vi "UI(Launcher).vi"(8 "error in":errorcluster) -> (0 "error out":errorcluster)   [LabVIEW 2017, in "UI.lvlib"]
doc: "The Queued Message Handler of a Worker."
uses:
  UI.lvlib
  <userlib>/_NEVSTOP/Communicable State Machine(CSM)/_Support/Priority Queue/Priority Queue.lvclass/Priority Queue.ctl
  _support/Settings.ctl
  Acquisition/_support/Hardware Configuration.ctl
  Acquisition/_support/Signal Type.ctl
  Logging/_support/Logging Configuration.ctl
  _support/Control Refs.ctl
  _support/UI State.ctl
  a36ec0c4-7f1b-4461-99c1-16b6f02c0371.vi
  1af51285-6659-428e-9c15-de70f1a207c9.vi
  1756710f-d813-4077-a3f9-6f06171a4225.vi
  242d01f8-d211-4c25-bb6c-8191a2acbe42.vi
  <userlib>/_NEVSTOP/Communicable State Machine(CSM)/_Polymophic/Add State(s) to Queue By BOOL(Element).vi
  <userlib>/_NEVSTOP/Communicable State Machine(CSM)/_Polymophic/Build No-Reply Asynchronous Message with Arguments.vi
  <userlib>/_NEVSTOP/Communicable State Machine(CSM)/_Support/CSMQ/_Obtain CSMQ.vi
  <userlib>/_NEVSTOP/Communicable State Machine(CSM)/_Support/FGV-BroadcastRegistry/Cache-Broadcast Registry Search Result.vi
  <userlib>/_NEVSTOP/Communicable State Machine(CSM)/_Support/CSMQ/_Create Resp Queue.vi
  <userlib>/_NEVSTOP/Communicable State Machine(CSM)/_Support/CSMQ/_Unlock CSMQ.vi
  <userlib>/_NEVSTOP/Communicable State Machine(CSM)/_Support/CSMQ/_Lock State CSMQ.vi
  <userlib>/_NEVSTOP/Communicable State Machine(CSM)/_Support/CSMQ/_Release CSMQ.vi
  <userlib>/_NEVSTOP/Communicable State Machine(CSM)/AdvanceAPI/CSM - Make String Arguments Safe.vi
  <userlib>/_NEVSTOP/Communicable State Machine(CSM)/addons/API-String-Arugments-Support/_Support/Query Data as API String Arguments(variant).vi
  <userlib>/_NEVSTOP/Communicable State Machine(CSM)/_Support/Message/Parse State with Arguments String.vi
  <userlib>/_NEVSTOP/Communicable State Machine(CSM)/_Support/CSMQ/_Input Name to CSM Mode.vi
  <userlib>/_NEVSTOP/Communicable State Machine(CSM)/_Support/Priority Queue/Not a Refnum.vi
  <userlib>/_NEVSTOP/Communicable State Machine(CSM)/Utility/uuid.vi
  <userlib>/_NEVSTOP/Communicable State Machine(CSM)/AdvanceAPI/CSM - Keywords.vi
  <userlib>/_NEVSTOP/Communicable State Machine(CSM)/_Support/GlobalEvent/FGV-GlobalEventRef.vi
  <userlib>/_NEVSTOP/Communicable State Machine(CSM)/_Support/CSMQ/_CSMQFGV.vi
  <userlib>/_NEVSTOP/Communicable State Machine(CSM)/_Support/CSMQ/_Dequeue CSMQ.vi
  <userlib>/_NEVSTOP/Communicable State Machine(CSM)/_Support/CSMQ/_Enqueue CSMQ.vi
  <userlib>/_NEVSTOP/Communicable State Machine(CSM)/_Support/GlobalEvent/FGV-StatusChangeEventRef.vi
  <userlib>/_NEVSTOP/Communicable State Machine(CSM)/_Support/FGV-BroadcastRegistry/global-Broadcast Cache Change Flag.vi
  <userlib>/_NEVSTOP/Communicable State Machine(CSM)/_Support/FGV-BroadcastRegistry/FGV-BroadcastRegistry.vi
  <userlib>/_NEVSTOP/Communicable State Machine(CSM)/addons/API-String-Arugments-Support/_Support/Data To API String Arguments.vi
  <userlib>/_NEVSTOP/Communicable State Machine(CSM)/addons/INI-Static-Variable-Support/LabVIEW-Config/Write Key (String).vi
  <userlib>/_NEVSTOP/Communicable State Machine(CSM)/addons/API-String-Arugments-Support/_Support/Convert API String Arguments to Data(variant).vi
  <userlib>/_NEVSTOP/Communicable State Machine(CSM)/addons/API-String-Arugments-Support/_Support/Data To SingleElementsArray_with_itself_csm.vi
  <userlib>/_NEVSTOP/Communicable State Machine(CSM)/addons/MassData-Parameter/_support/FGV-MassData.vi
  _support/Settings Dialog.vi
  Acquisition/Acquisition.lvlib
  Logging/Logging.lvlib
  <userlib>/_NEVSTOP/Communicable State Machine(CSM)/Communicable State Machine.lvlib
  <userlib>/_NEVSTOP/Communicable State Machine(CSM)/addons/MassData-Parameter/CSM MassData Parameter Support.lvlib
  <userlib>/_NEVSTOP/Communicable State Machine(CSM)/addons/INI-Static-Variable-Support/INI-Static-Variable-Support.lvlib
  <userlib>/_NEVSTOP/Communicable State Machine(CSM)/addons/INI-Static-Variable-Support/LabVIEW-Config/LabVIEW-Config.lvlib
  Algorithm/Algorithm.lvlib
panel:
  out "State History":string
  out "Data":waveform(dbl)[](graph)
  in  "Settings":bool
  in  "Start":bool
  in  "Stop":bool
  out "Status":string
  in  "Exit":bool
  # "Continuous Measurement and Data Logger - CSM Version"
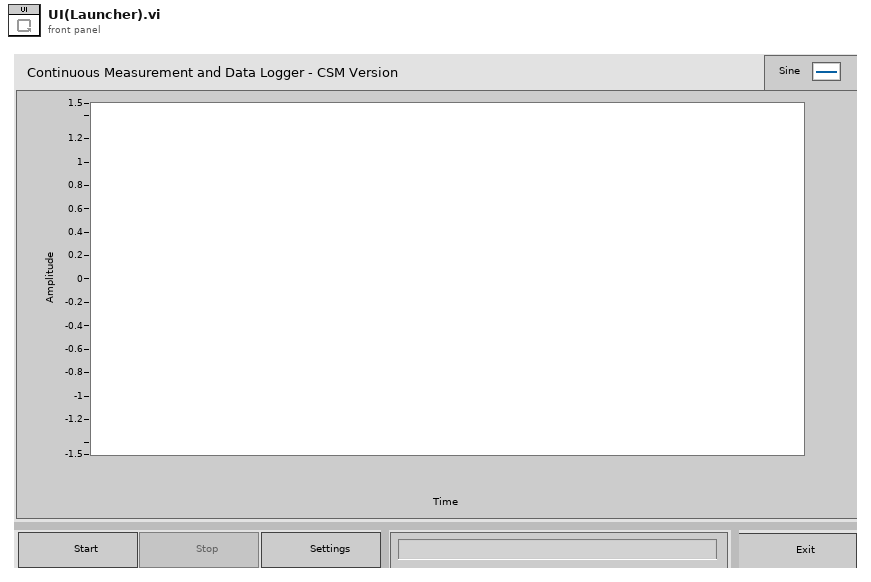
[diagram p1: front panel]
types:
  T1 = enum32{"Invalid", "Standard", "Closed", "Hidden", "Minimized", "Maximized"}
  T2 = enum32{"invalid app kind", "Development System", "Run Time System", "Student Edition", "Embedded LabVIEW", "Evaluation", "Custom"}
  T3 = typedef "UI.lvlib/UI State.ctl" = enum16{"Idle", "Acquiring and Logging", "Waiting for Exit", "Waiting for Exit (Acq Stopped)", "Waiting for Exit (Log Stopped)", "Waiting for Stop", "Waiting for Stop (Acq Stopped)", "Waiting for Stop (Log Stopped)"}
  T4 = typedef "UI.lvlib/Settings.ctl" = cluster{"Hardware":T5, "Logging":T7}
  T5 = typedef "Acquisition.lvlib/Hardware Configuration.ctl" = cluster{"Resource":string, "SignalType":T6}
  T6 = typedef "Acquisition.lvlib/Signal Type.ctl" = enum16{"Sine Wave", "Square with Noise"}
  T7 = typedef "Logging.lvlib/Logging Configuration.ctl" = cluster{"BasePath":path}
  T8 = typedef "UI.lvlib/Control Refs.ctl" = cluster{"Start Ref":refnum<vi>, "Stop Ref":refnum<vi>, "Settings Ref":refnum<vi>, "Exit Ref":refnum<vi>, "Status Ref":refnum<vi>, "Data Ref":refnum<vi>}
  T9 = cluster{"Core":cluster{"Current VI Reference":refnum<vi>, "Close Panel on Exit?":bool}, "Config":T4, "UI Refs":T8, "State":T3}
  T10 = cluster{"Current VI Reference":refnum<vi>, "Close Panel on Exit?":bool}
  T11 = typedef "LabVIEW-Config.lvlib/Config.ctl" = cluster{"Path":path, "Lines":string[], "Tokens":enum8{"comment", "section", "key"}[], "Modified?":bool}
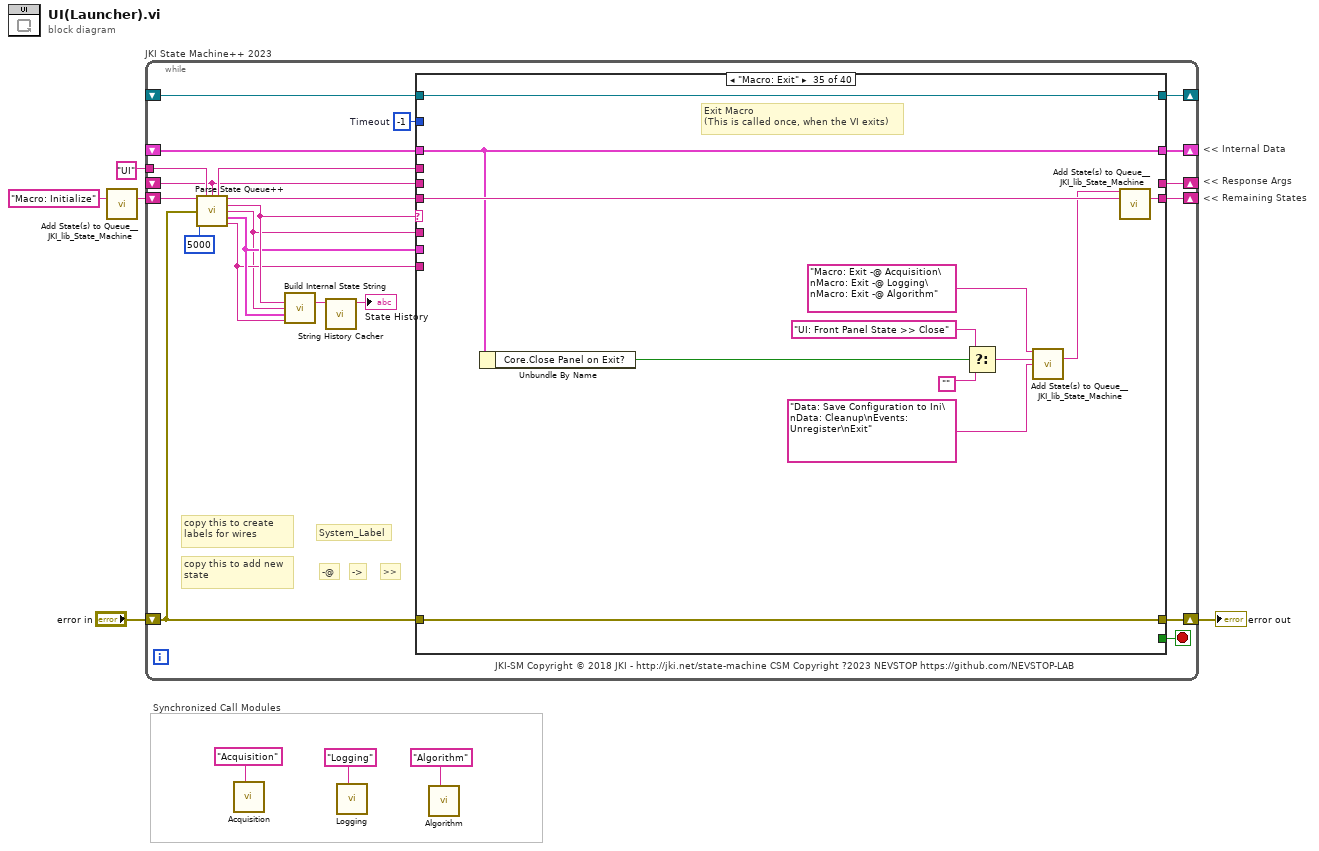
[diagram p0: block diagram]
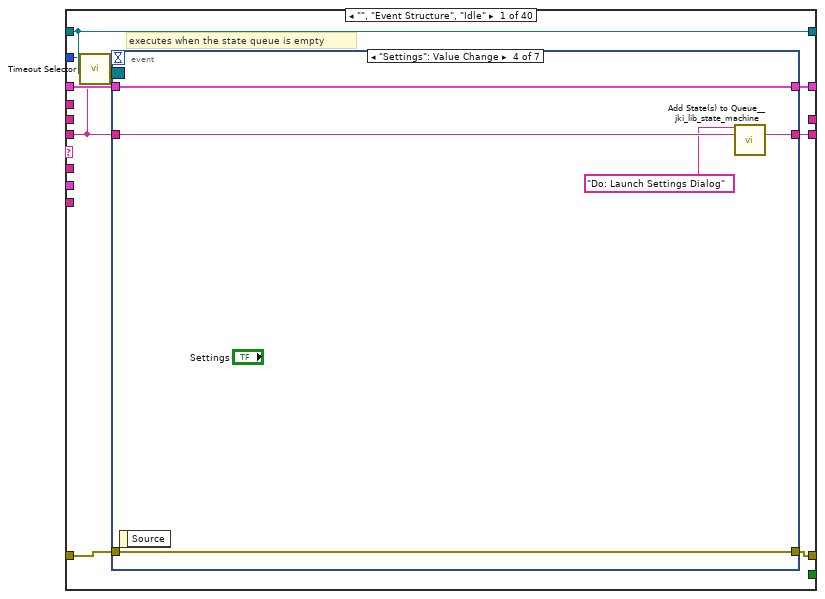
[diagram p2: hidden frame]
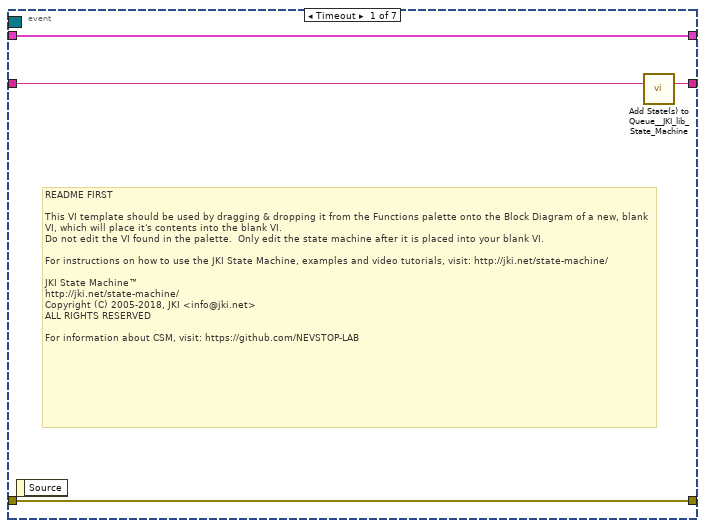
[diagram p3: hidden frame]
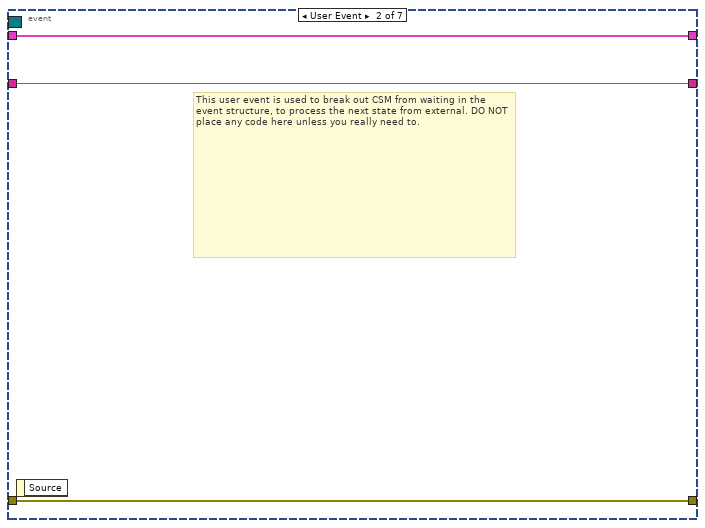
[diagram p4: hidden frame]
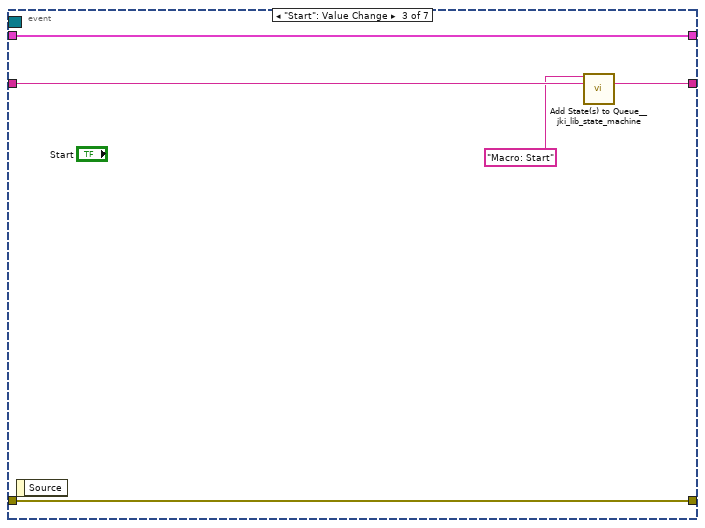
[diagram p5: hidden frame]
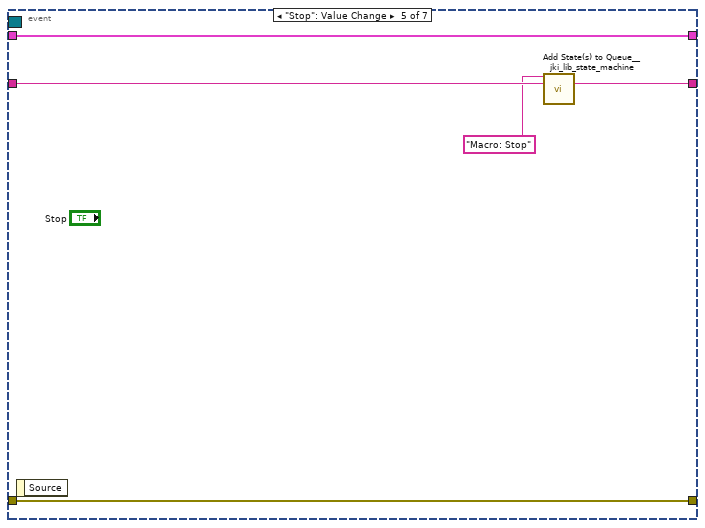
[diagram p6: hidden frame]
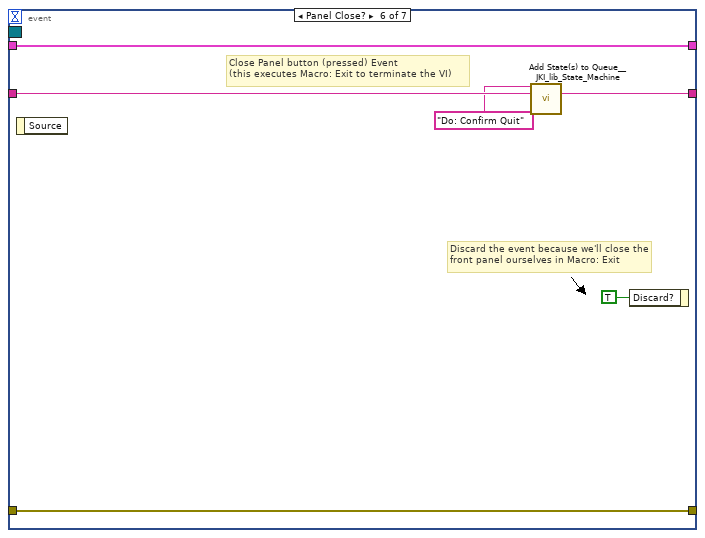
[diagram p7: hidden frame]
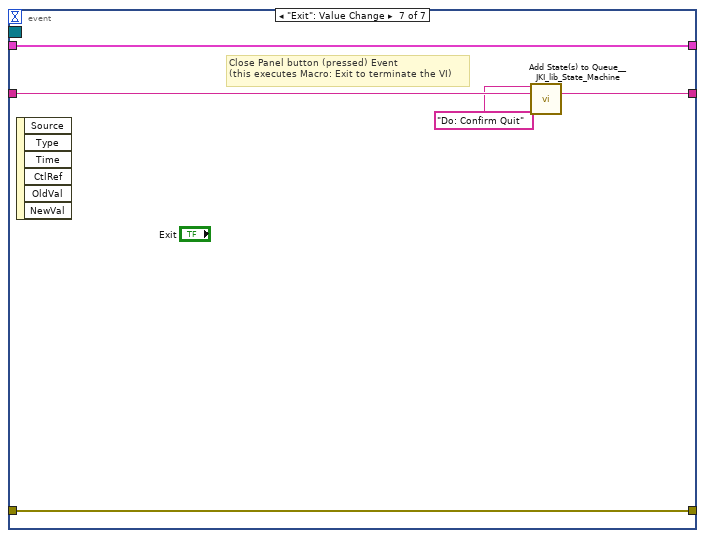
[diagram p8: hidden frame]
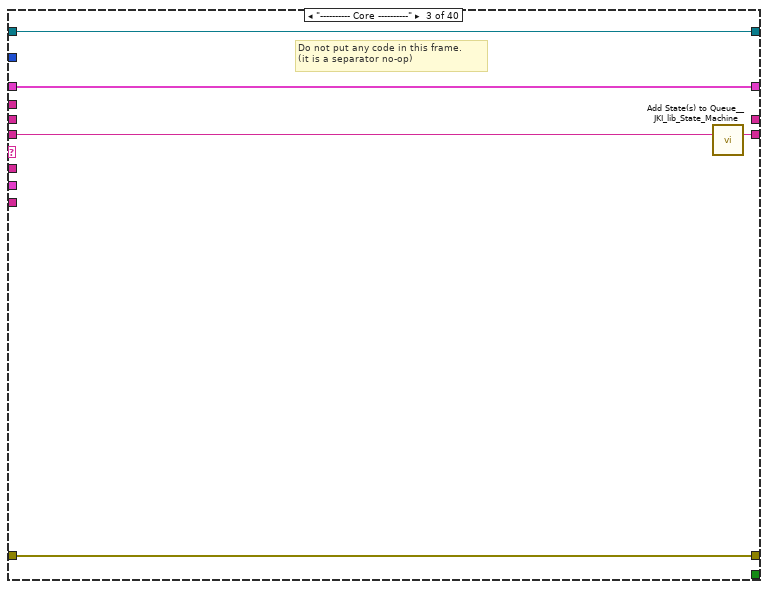
[diagram p10: hidden frame]
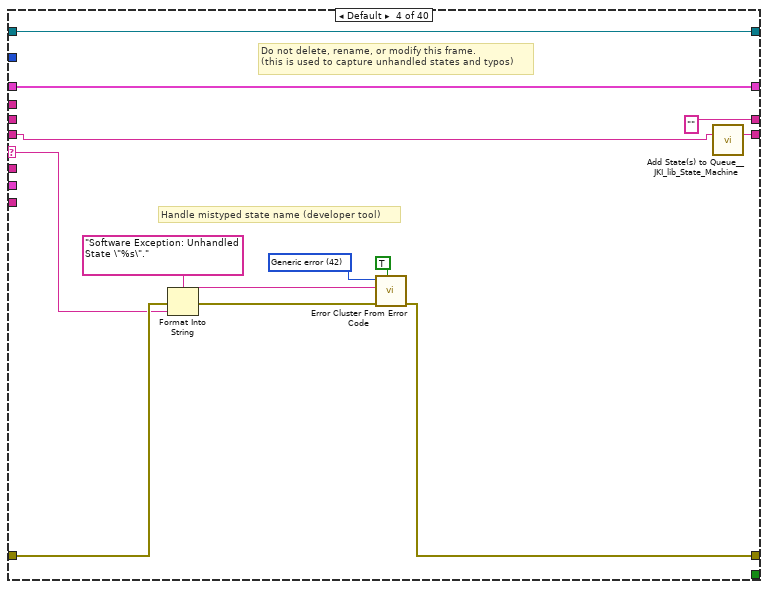
[diagram p11: hidden frame]
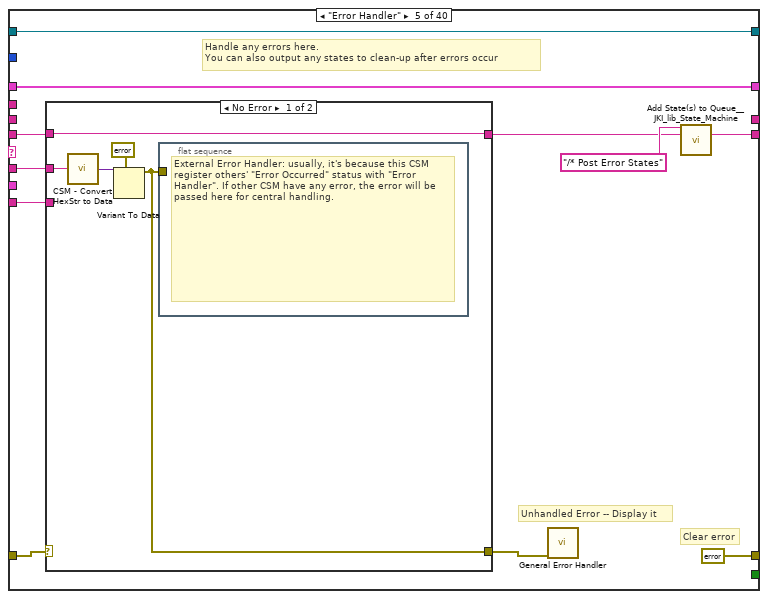
[diagram p12: hidden frame]
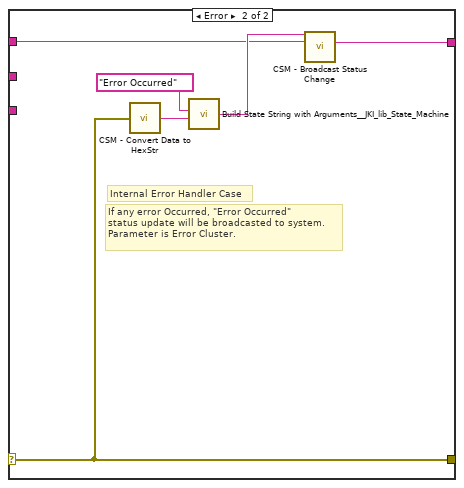
[diagram p13: hidden frame]
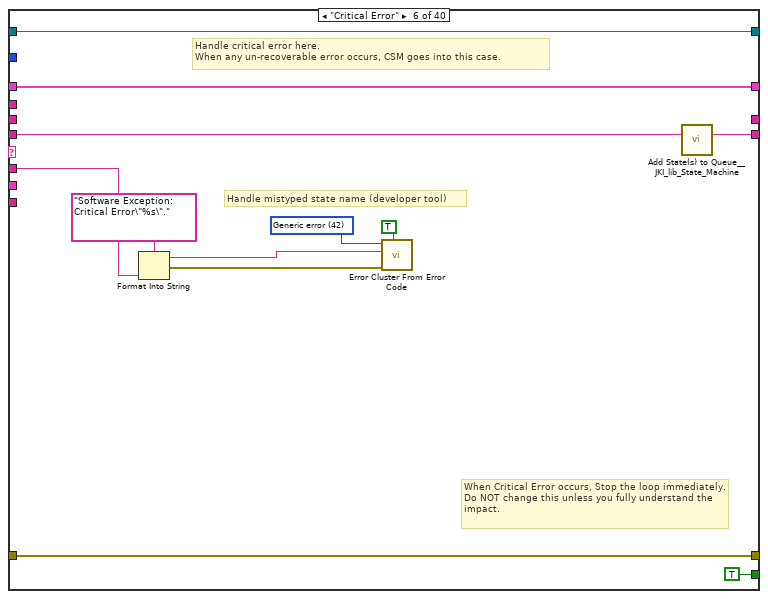
[diagram p14: hidden frame]
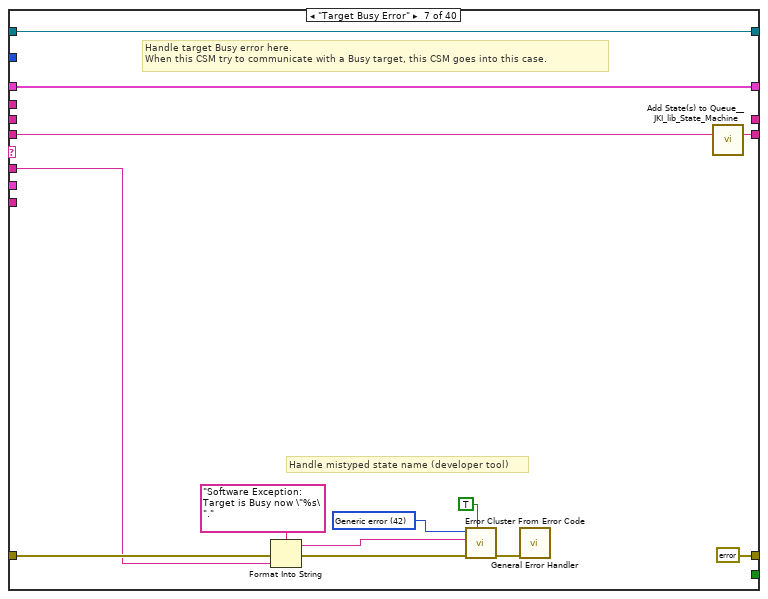
[diagram p15: hidden frame]
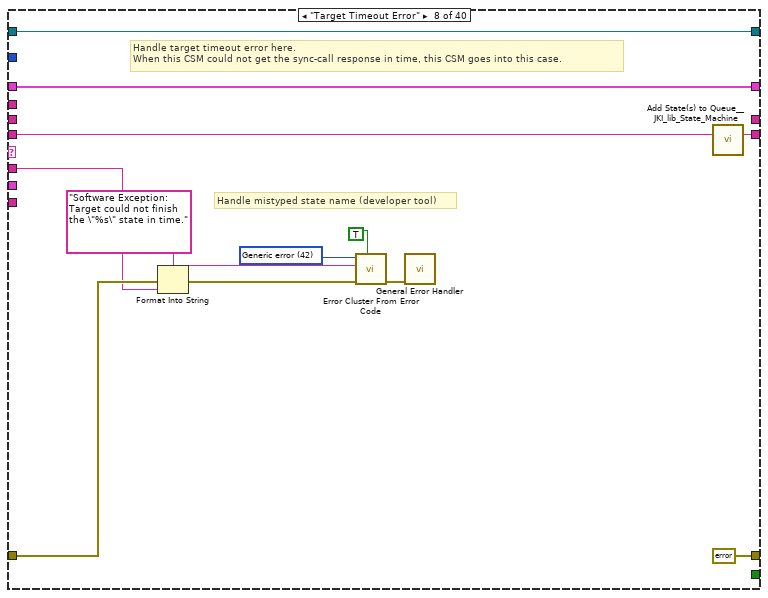
[diagram p16: hidden frame]
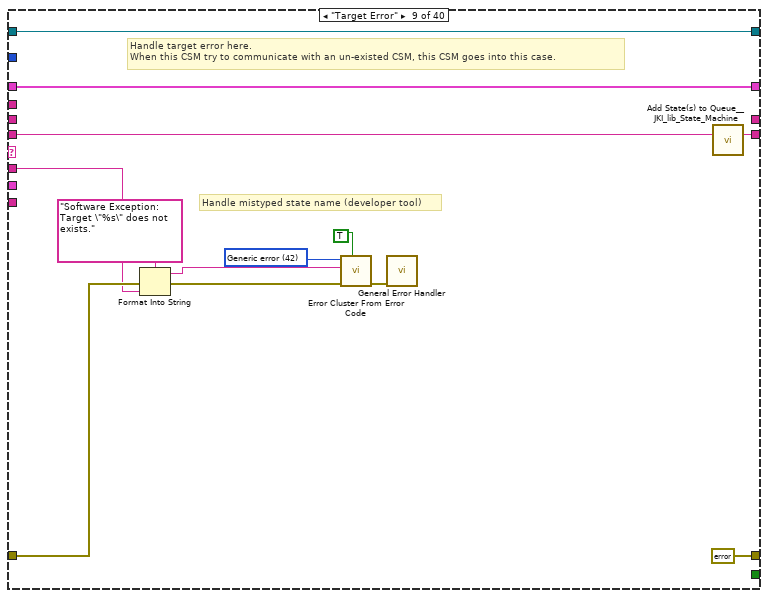
[diagram p17: hidden frame]
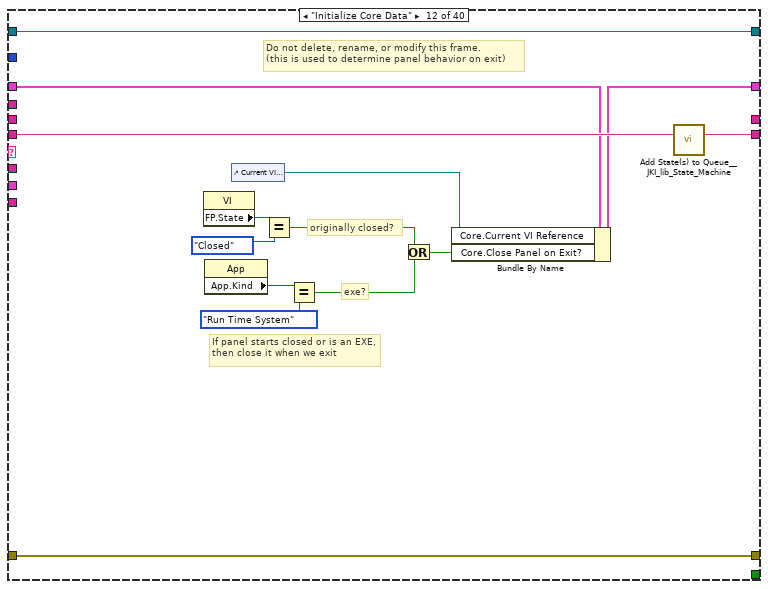
[diagram p20: hidden frame]
diagram:
  # "Synchronized Call Modules"
  # "<< Internal Data"
  # "<< Response Args"
  # "<< Remaining States"
  n1 = call <vilib>:"Add State(s) to Queue__JKI_lib_State_Machine.vi"("State(s) in (\"\")"="Macro: Initialize") -> ("States Out"=w6:string)  [unwired: 14 in]
  n2 = while "JKI State Machine++ 2023" {
    shift-right: [w25] -> _
    shift-left: _ -> [w24]
    shift-right: [w28] -> w4
    shift-left: "error in" -> [w22]
    shift-right: [w27] -> _
    shift-left: w6 -> [w29]
    tunnel: "UI" ("Name(\"\" to use uuid)") -> [w17]
    shift-right: [w20] -> _
    shift-left: _ -> [w10]
    shift-right: [w19] -> _
    shift-left: _ -> [w18]
    stop <- w26 stop-if-true
    w23 = -1  # Timeout
    # "JKI-SM Copyright © 2018 JKI - http://jki.net/state-machine CSM Copyright ?2023 NEVSTOP https://github.com/NEVSTOP-LAB"
    # "copy this to add new state"
    # ">>"
    # "->"
    # "-@"
    # "copy this to create labels for wires"
    # "System_Label"
    n3 = call <userlib>:"Parse State Queue++.vi"("State Queue"=w29, "Name(\"\" to use uuid)"=w17, "Response Arguments"=w10, "Error In (no error)"=w22, "Response Timeout(5000ms)"=5000 ("Response Timeout(1000ms)")) -> ("Name Used"=w11:string, "Remaining States"=w30:string, "Current State"=w14:string, "Arguments"=w9:string, ">> Response Source Message >>"=w13:cluster{"State":string, "Arguments":string}, ">> Source CSM >>"=w12:string)  [unwired: 5 in]
    n4 = call <userlib>:"Build Internal State String.vi"("State"=w14, "Arguments (\"\")"=w9, ">> Response Source Message >>"=w13, "Source (\"\")"=w12) -> ("State with Arguments"=w15:string)  [unwired: 11 in]
    n5 = call <userlib>:"String History Cacher.vi"("String"=w15) -> ("String Cache"=→"State History":string)  [unwired: 10 in]
    n6 = case shown="\"Macro: Exit\"" w14 {
      selector: w14 -> [_ _ _ w84 _ _ _ _ _ _ _ _ _ _ _ _ _ _ _ _ _ _ _ _ _ _ _ _ _ _ _ _ _ _ _ _ _ _ _ _]
      tunnel: w30 -> [w31 w75 w81 w88 w98 w126 w131 w149 w162 w170 w174 w189 w196 w201 w216 w220 w240 w258 w265 w272 w277 w283 w287 w293 w310 w321 w333 w341 w357 w429 w434 w441 w447 w462 w483 w488 w494 w505 w517 w532]
      tunnel: w9 -> [_ _ _ _ w96 w119 w133 w145 w158 _ _ _ _ _ _ _ _ w256 w262 _ _ _ _ _ _ _ _ w336 w351 w426 _ _ _ _ _ _ w489 _ _ _]
      tunnel: w24 -> [w38 w74 w78 w86 w104 w127 w135 w147 w160 w169 w173 w182 w194 w198 _ w222 w232 w255 w263 w267 w274 w282 w286 w290 w296 w311 w323 w339 w353 w428 w431 w438 w450 w458 w480 w485 w491 w500 w516 w527]
      tunnel: [w37 w76 w79 w90 errorcluster {"status"=FALSE, "code"=0, "source"=""} ("error out") w128 errorcluster {"status"=FALSE, "code"=0, "source"=""} ("error out") errorcluster {"status"=FALSE, "code"=0, "source"=""} ("error out") errorcluster {"status"=FALSE, "code"=0, "source"=""} ("error out") w171 w175 w186 w193 w199 w202 w223 w241 w253 w261 w268 w275 w278 w285 w291 w308 w322 w334 w337 w354 w423 w432 w439 w453 w466 w481 w486 w492 w497 w520 w525] -> w28
      tunnel: w22 -> [w36 w76 w79 w89 w102 w128 w137 w150 w163 w171 w175 w186 w193 w199 w203 w223 w241 _ _ w269 w275 _ w288 w291 w308 w322 w334 w338 w355 _ w432 w439 w453 w466 w481 w486 w492 w498 w520 w526]
      tunnel: [w39 w75 w80 w87 w100 w125 w136 w148 w161 w170 w174 w188 w195 w200 w215 w219 w240 w258 w265 w271 w276 w283 w287 w292 w309 w321 w333 w340 w356 w429 w433 w440 w448 w463 w482 w487 w493 w504 w518 w523] -> w27
      tunnel: [_ _ _ _ _ TRUE _ _ _ _ _ _ TRUE _ _ _ _ _ _ _ _ _ _ _ _ _ _ _ _ _ _ _ _ _ _ _ _ _ _ _] -> w26
      tunnel: [w35 w74 w78 w86 w104 w127 w135 w147 w160 w169 w173 w187 w194 w198 w214 w222 w232 w254 w259 w267 w274 w282 w286 w290 w295 w311 w323 w339 w353 w428 w431 w438 w449 w464 w480 w485 w491 w499 w516 w524] -> w25
      tunnel: w23 -> [w33 _ _ _ _ _ _ _ _ _ _ _ _ _ _ _ _ _ _ _ _ _ _ _ _ _ _ _ _ _ _ _ _ _ _ _ _ _ _ _]
      tunnel: w12 -> [_ _ _ _ w95 _ _ _ _ _ _ _ _ _ _ _ _ _ _ _ _ _ _ _ _ _ _ _ _ _ _ _ _ _ _ _ _ _ _ _]
      tunnel: w13 -> [_ _ _ _ _ _ _ _ _ _ _ _ _ _ _ _ _ _ _ _ _ _ _ _ _ _ _ _ _ _ _ _ _ _ _ _ _ _ _ _]
      tunnel: [_ _ _ "" _ _ _ _ _ _ _ _ _ _ _ _ _ _ w260 _ _ _ _ _ _ _ _ _ _ _ _ _ _ _ _ _ _ _ _ _] -> w20
      tunnel: [w34 w73 w77 w82 w103 w117 w132 w144 w157 w168 w172 w176 w191 w197 w212 w221 w239 w257 w264 w266 w273 w281 w284 w289 w307 w320 w332 w335 w350 w427 w430 w437 w452 w465 w473 w484 w490 w503 w519 w531] -> w19
      tunnel: w18 -> [w34 w73 w77 w82 w103 w117 w132 w144 w157 w168 w172 w176 w191 w197 w212 w221 w239 w257 w264 w266 w273 _ w284 w289 w307 w320 w332 w335 w350 w427 w430 w437 w452 w465 w473 w484 w490 w503 w519 w531]
      tunnel: w11 -> [_ _ _ _ _ _ _ _ _ _ _ _ _ _ _ _ _ _ _ _ _ w280 _ _ _ _ _ _ _ _ _ _ _ _ _ _ _ _ _ _]
      tunnel: w10 -> [_ _ _ _ _ _ _ _ _ _ _ _ _ _ _ _ _ _ _ _ _ _ _ _ _ _ _ _ _ _ _ _ _ _ _ _ _ _ _ _]
      frame "", "Event Structure", "Idle" {
        # "executes when the state queue is empty"
        n7 = call <userlib>:"Timeout Selector.vi"("Remaining States"=w31, "Timeout Expected"=w33) -> ("Timeout"=w32:i32)  [unwired: 5 in]
        n8 = event shown="[3] \"Settings\": Value Change" {
          selector: w34 -> [_ _ _ _ _ _ _]
          dyn-events: _ -> [_ _ _ _ _ _ _]
          timeout: w32 -> [_ _ _ _ _ _ _]
          tunnel: w31 -> [w43 w45 w48 w53 w58 w67 w72]
          tunnel: [w42 w45 w49 w54 w59 w66 w71] -> w39
          tunnel: w38 -> [w40 w46 w50 w55 w60 w64 w69]
          tunnel: [w41 w44 w51 w56 w61 w65 w70] -> w37
          tunnel: w36 -> [w41 w44 w51 w56 w61 w65 w70]
          tunnel: [w40 w46 w50 w55 w60 w64 w69] -> w35
          event Timeout {
            # "README FIRST\n \nThis VI template should be used by dragging & dropping it from the Functions palette onto the Block Diagram of a new, blank VI, which will place it's contents into the blank VI. \nDo not edit the VI found in the palette.  Only edit the state machine after it is placed into your blank VI.\n \nFor instructions on how to use the JKI State Machine, examples and video tutorials, visit: http://jki.net/state-machine/\n\nJKI State Machine™\nhttp://jki.net/state-machine/\nCopyright (C) 2005-2018, JKI <info@jki.net>\nALL RIGHTS RESERVED\n\nFor information about CSM, visit: https://github.com/NEVSTOP-LAB"
            n9 = event-data() -> ()  [unwired: 1 in, 1 out]
            n10 = call <vilib>:"Add State(s) to Queue__JKI_lib_State_Machine.vi"("State(s) in (\"\")"=w43) -> ("States Out"=w42:string)  [unwired: 14 in]
          }
          event User Event {
            # "This user event is used to break out CSM from waiting in the event structure, to process the next state from external. DO NOT place any code here unless you really need to."
            n11 = event-data() -> ()  [unwired: 1 in, 1 out]
          }
          event "Start": Value Change {
            n12 = event-data() -> ()  [unwired: 1 in, 1 out]
            n13 = call <vilib>:"Add State(s) to Queue__jki_lib_state_machine.vi"("State(s) in Front (\"\")"="Macro: Start" ("State(s) in Front (\"\")"), "State(s) in (\"\")"=w48) -> ("States Out"=w49:string)  [unwired: 13 in]
          }
          event "Settings": Value Change {
            n14 = event-data() -> ()  [unwired: 1 in, 1 out]
            n15 = call <vilib>:"Add State(s) to Queue__jki_lib_state_machine.vi"("State(s) in Front (\"\")"="Do: Launch Settings Dialog" ("State(s) in Front (\"\")"), "State(s) in (\"\")"=w53) -> ("States Out"=w54:string)  [unwired: 13 in]
          }
          event "Stop": Value Change {
            n16 = event-data() -> ()  [unwired: 1 in, 1 out]
            n17 = call <vilib>:"Add State(s) to Queue__jki_lib_state_machine.vi"("State(s) in Front (\"\")"="Macro: Stop" ("State(s) in Front (\"\")"), "State(s) in (\"\")"=w58) -> ("States Out"=w59:string)  [unwired: 13 in]
          }
          event Panel Close? {
            # "Discard the event because we'll close the front panel ourselves in Macro: Exit"
            # "Close Panel button (pressed) Event\n(this executes Macro: Exit to terminate the VI)"
            n18 = event-data() -> ()  [unwired: 1 in, 1 out]
            n19 = call <vilib>:"Add State(s) to Queue__JKI_lib_State_Machine.vi"("State(s) in Front (\"\")"="Do: Confirm Quit", "State(s) in (\"\")"=w67) -> ("States Out"=w66:string)  [unwired: 13 in]
            n20 = event-data("Discard?"=TRUE) -> ()  [unwired: 1 in, 1 out]
          }
          event "Exit": Value Change {
            # "Close Panel button (pressed) Event\n(this executes Macro: Exit to terminate the VI)"
            n21 = event-data() -> ()  [unwired: 1 in, 6 out]
            n22 = call <vilib>:"Add State(s) to Queue__JKI_lib_State_Machine.vi"("State(s) in Front (\"\")"="Do: Confirm Quit", "State(s) in (\"\")"=w72) -> ("States Out"=w71:string)  [unwired: 13 in]
          }
        }
      }
      frame "CSM Documentation" {
        # "CSM Documentation"
        # "State Syntax:\nStateCategory: State >> Argument -@ CSMName\nStateCategory: State >> Argument -> CSMName\n\nLine Terminator: Line feed"
        # "Commenting:\nTo add a comment use \"//\" or \"#\" and all text to the right will be ignored\nCommenting Example:\nUI: Initialize // This initializes the UI\n// Another comment line"
        # "Example:\nUI: Help >> About -@Main\nUI: Help >> About ->Main\n\nWhere \"UI\" is the state category\nWhere \"Help\" is the state\nWhere \"About\" is the argument\nWhere \"Main\" is the Name of CSM,which actually run the \"UI: Help >> About\"\n\n    \"-@\" stands for sync state. Current CSM will wait until the state is finished. \n            - if \"Main\" named CSM does not exist, \"Target Error\" will occur.\n            - if \"Main\" named CSM is in another sync remote state, \"Target Busy Error\" will occur.\n            - if \"Main\" named CSM could not finish the state in time, \"Target Timeout Error\" will occur.\n            - if everything is right. \"Response\" will occur with Argument back from \"Main\" named CSM. \n\n    \"->\" stands for async state. Current CSM will post the state and continue to next state in next iteration.\n            - if \"Main\" named CSM does not exist, \"Target Error\" will occur.\n            - if everything is right. \"Async Message Posted\" will occur.\n            - After State is finished. Caller will receive a \"Async Response\" state from callee.\n\nWhen duplicated name is used for multiple CSM module or some framework problem happens, \"Critical Error\" will occur."
      }
      frame "---------- Core ----------" {
        # "Do not put any code in this frame.\n(it is a separator no-op)"
        n23 = call <vilib>:"Add State(s) to Queue__JKI_lib_State_Machine.vi"("State(s) in (\"\")"=w81) -> ("States Out"=w80:string)  [unwired: 14 in]
      }
      frame Default {
        w93 = 42 items=["No error", "Argument error", "Memory is full", "Out of zone", "End of file", "File already open", "Generic file I/O error", "File not found", "File permission error", "Disk is full", "Duplicate path", "Too many files open", "System feature not enabled", "Resource file not found", "Cannot add resource", "Resource not found", "Image not found", "Image memory error", "Pen does not exist", "Config type invalid", "Config token not found", "Config parse error", "Config memory error", "Bad external code format", "Bad external code offset", "External code not present", "Null window", "Destroy window error", "Null menu", "Print aborted", "Bad print record", "Print driver error", "Windows error during printing", "Memory error during printing", "Print dialog error", "Generic print error", "Invalid device refnum", "Device not found", "Device parameter error", "Device unit error", "Cannot open device", "Device call aborted", "Generic error", "Cancelled by user", "Object ID too low", "Object ID too high", "Object not in heap", "Unknown heap", "Unknown object (invalid DefProc)", "Unknown object (DefProc not in table)", "Message out of range", "Invalid (null) method", "Unknown message", "Manager call not supported", "Bad address", "Network operation in progress", "Network operation timed out", "Connection is busy", "Network attribute not supported", "Network error", "Address in use", "System out of memory", "Connection aborted", "Connection refused", "Not connected", "Already connected", "Connection closed", "Initialization error (interapplication manager)", "Bad occurrence", "Wait on unbound occurrence handler", "Occurrence queue overflow", "Datalog type conflict", "Unused", "Unrecognized type (interapplication manager)", "Memory corrupt", "Failed to make temporary DLL", "Old CIN version", "Drag socket not found", "Failed to load drop-object", "Failed to register OLE object", "Failed to release OLE object", "Format specifier type mismatch", "Unknown format specifier", "Too few format specifiers", "Too many format specifiers", "Scan failed", "Newer CIN version", "Error converting to variant", "Runtime menu error", "Password tampered", "Variant attribute not found", "Incompatible variant data type", "Event data is not available", "Event Store is not present", "Occurrence is not found", "Event Queue is not created", "Event info is not available", "Refnum passed is NULL", "Error retrieving Class GUID", "Error retrieving CoClass GUID", "Error retrieving TypeLib GUID.", "Bad built application magic bytes.", "Specific driver is different from the specific driver associated with the Logical Name.", "There is no session opened to the class driver.", "Max Error", "MAX - Error with config objects", "MAX - Error loading configuration", "MAX - Group not supported"]
        # "Do not delete, rename, or modify this frame.\n(this is used to capture unhandled states and typos)"
        # "Handle mistyped state name (developer tool)"
        n24 = Format Into String(format string="Software Exception: Unhandled State \"%s\"." ("message"), error in=w89, w84) -> (resulting string=w92:string, error out=w91:errorcluster)  [unwired: 1 in]
        n25 = call <vilib>:"Error Cluster From Error Code.vi"("show call chain? (False)"=TRUE, "error in (no error)"=w91, "error message (\"\")"=w92, "error code (0)"=w93) -> ("error out"=w90:errorcluster)  [unwired: 5 in]
        n26 = call <vilib>:"Add State(s) to Queue__JKI_lib_State_Machine.vi"("State(s) in (\"\")"=w88) -> ("States Out"=w87:string)  [unwired: 14 in]
      }
      frame "Error Handler" {
        # "Unhandled Error -- Display it"
        # "Handle any errors here.\nYou can also output any states to clean-up after errors occur"
        # "Clear error"
        n27 = case shown="No Error" w102 {
          selector: w102 -> [_ w111]
          tunnel: [w107 w113] -> w99
          tunnel: w98 -> [w107 w112]
          tunnel: [w106 w111] -> w97
          tunnel: w96 -> [w108 _]
          tunnel: w95 -> [_ _]
          frame No Error {
            n28 = call <userlib>:"CSM - Convert HexStr to Data.vi"("HEX String"=w108) -> ("Variant"=w110:variant)  [unwired: 7 in, 1 out]
            n29 = Variant To Data(type=errorcluster {"status"=FALSE, "code"=0, "source"=""} ("error in (no error)"), Variant=w110) -> (data=w106:errorcluster)  [unwired: 1 in, 1 out]
            n30 = flat-sequence {
              tunnel: w106 -> [_]
              frame #0 {
                # "External Error Handler: usually, it's because this CSM register others' \"Error Occurred\" status with \"Error Handler\". If other CSM have any error, the error will be passed here for central handling."
              }
            }
          }
          frame Error {
            # "Internal Error Handler Case"
            # "If any error Occurred, \"Error Occurred\" \nstatus update will be broadcasted to system.\nParameter is Error Cluster."
            n31 = call <userlib>:"CSM - Convert Data to HexStr.vi"("Variant"=w111) -> ("HEX String (0-9,A-F)"=w115:string)  [unwired: 8 in]
            n32 = call <vilib>:"Build State String with Arguments__JKI_lib_State_Machine.vi"("Arguments (\"\")"=w115, "State"="Error Occurred" ("Status with Arguments")) -> ("State with Arguments"=w114:string)  [unwired: 4 in]
            n33 = call <userlib>:"CSM - Broadcast Status Change.vi"("Status with Arguments"=w114, "State Queue"=w112) -> ("Remaining States"=w113:string)  [unwired: 13 in]
          }
        }
        n34 = call <vilib>:"General Error Handler.vi"("error in (no error)"=w97) -> ()  [unwired: 10 in, 5 out]
        n35 = call <vilib>:"Add State(s) to Queue__JKI_lib_State_Machine.vi"("State(s) in Front (\"\")"="/* Post Error States", "State(s) in (\"\")"=w99) -> ("States Out"=w100:string)  [unwired: 13 in]
      }
      frame "Critical Error" {
        w123 = 42 items=["No error", "Argument error", "Memory is full", "Out of zone", "End of file", "File already open", "Generic file I/O error", "File not found", "File permission error", "Disk is full", "Duplicate path", "Too many files open", "System feature not enabled", "Resource file not found", "Cannot add resource", "Resource not found", "Image not found", "Image memory error", "Pen does not exist", "Config type invalid", "Config token not found", "Config parse error", "Config memory error", "Bad external code format", "Bad external code offset", "External code not present", "Null window", "Destroy window error", "Null menu", "Print aborted", "Bad print record", "Print driver error", "Windows error during printing", "Memory error during printing", "Print dialog error", "Generic print error", "Invalid device refnum", "Device not found", "Device parameter error", "Device unit error", "Cannot open device", "Device call aborted", "Generic error", "Cancelled by user", "Object ID too low", "Object ID too high", "Object not in heap", "Unknown heap", "Unknown object (invalid DefProc)", "Unknown object (DefProc not in table)", "Message out of range", "Invalid (null) method", "Unknown message", "Manager call not supported", "Bad address", "Network operation in progress", "Network operation timed out", "Connection is busy", "Network attribute not supported", "Network error", "Address in use", "System out of memory", "Connection aborted", "Connection refused", "Not connected", "Already connected", "Connection closed", "Initialization error (interapplication manager)", "Bad occurrence", "Wait on unbound occurrence handler", "Occurrence queue overflow", "Datalog type conflict", "Unused", "Unrecognized type (interapplication manager)", "Memory corrupt", "Failed to make temporary DLL", "Old CIN version", "Drag socket not found", "Failed to load drop-object", "Failed to register OLE object", "Failed to release OLE object", "Format specifier type mismatch", "Unknown format specifier", "Too few format specifiers", "Too many format specifiers", "Scan failed", "Newer CIN version", "Error converting to variant", "Runtime menu error", "Password tampered", "Variant attribute not found", "Incompatible variant data type", "Event data is not available", "Event Store is not present", "Occurrence is not found", "Event Queue is not created", "Event info is not available", "Refnum passed is NULL", "Error retrieving Class GUID", "Error retrieving CoClass GUID", "Error retrieving TypeLib GUID.", "Bad built application magic bytes.", "Specific driver is different from the specific driver associated with the Logical Name.", "There is no session opened to the class driver.", "Max Error", "MAX - Error with config objects", "MAX - Error loading configuration", "MAX - Group not supported"]
        # "Handle critical error here.\nWhen any un-recoverable error occurs, CSM goes into this case."
        # "When Critical Error occurs, Stop the loop immediately. Do NOT change this unless you fully understand the impact."
        # "Handle mistyped state name (developer tool)"
        n36 = Format Into String(format string="Software Exception: Critical Error\"%s\"." ("message"), w119) -> (resulting string=w122:string, error out=w121:errorcluster)  [unwired: 2 in]
        n37 = call <vilib>:"Error Cluster From Error Code.vi"("show call chain? (False)"=TRUE, "error in (no error)"=w121, "error message (\"\")"=w122, "error code (0)"=w123) -> ()  [unwired: 5 in, 1 out]
        n38 = call <vilib>:"Add State(s) to Queue__JKI_lib_State_Machine.vi"("State(s) in (\"\")"=w126) -> ("States Out"=w125:string)  [unwired: 14 in]
      }
      frame "Target Busy Error" {
        w140 = 42 items=["No error", "Argument error", "Memory is full", "Out of zone", "End of file", "File already open", "Generic file I/O error", "File not found", "File permission error", "Disk is full", "Duplicate path", "Too many files open", "System feature not enabled", "Resource file not found", "Cannot add resource", "Resource not found", "Image not found", "Image memory error", "Pen does not exist", "Config type invalid", "Config token not found", "Config parse error", "Config memory error", "Bad external code format", "Bad external code offset", "External code not present", "Null window", "Destroy window error", "Null menu", "Print aborted", "Bad print record", "Print driver error", "Windows error during printing", "Memory error during printing", "Print dialog error", "Generic print error", "Invalid device refnum", "Device not found", "Device parameter error", "Device unit error", "Cannot open device", "Device call aborted", "Generic error", "Cancelled by user", "Object ID too low", "Object ID too high", "Object not in heap", "Unknown heap", "Unknown object (invalid DefProc)", "Unknown object (DefProc not in table)", "Message out of range", "Invalid (null) method", "Unknown message", "Manager call not supported", "Bad address", "Network operation in progress", "Network operation timed out", "Connection is busy", "Network attribute not supported", "Network error", "Address in use", "System out of memory", "Connection aborted", "Connection refused", "Not connected", "Already connected", "Connection closed", "Initialization error (interapplication manager)", "Bad occurrence", "Wait on unbound occurrence handler", "Occurrence queue overflow", "Datalog type conflict", "Unused", "Unrecognized type (interapplication manager)", "Memory corrupt", "Failed to make temporary DLL", "Old CIN version", "Drag socket not found", "Failed to load drop-object", "Failed to register OLE object", "Failed to release OLE object", "Format specifier type mismatch", "Unknown format specifier", "Too few format specifiers", "Too many format specifiers", "Scan failed", "Newer CIN version", "Error converting to variant", "Runtime menu error", "Password tampered", "Variant attribute not found", "Incompatible variant data type", "Event data is not available", "Event Store is not present", "Occurrence is not found", "Event Queue is not created", "Event info is not available", "Refnum passed is NULL", "Error retrieving Class GUID", "Error retrieving CoClass GUID", "Error retrieving TypeLib GUID.", "Bad built application magic bytes.", "Specific driver is different from the specific driver associated with the Logical Name.", "There is no session opened to the class driver.", "Max Error", "MAX - Error with config objects", "MAX - Error loading configuration", "MAX - Group not supported"]
        # "Handle target Busy error here.\nWhen this CSM try to communicate with a Busy target, this CSM goes into this case."
        # "Handle mistyped state name (developer tool)"
        n39 = Format Into String(format string="Software Exception: Target is Busy now \"%s\"." ("message"), error in=w137, w133) -> (resulting string=w139:string, error out=w138:errorcluster)  [unwired: 1 in]
        n40 = call <vilib>:"Error Cluster From Error Code.vi"("show call chain? (False)"=TRUE, "error in (no error)"=w138, "error message (\"\")"=w139, "error code (0)"=w140) -> ("error out"=w130:errorcluster)  [unwired: 5 in]
        n41 = call <vilib>:"General Error Handler.vi"("error in (no error)"=w130) -> ()  [unwired: 10 in, 5 out]
        n42 = call <vilib>:"Add State(s) to Queue__JKI_lib_State_Machine.vi"("State(s) in (\"\")"=w131) -> ("States Out"=w136:string)  [unwired: 14 in]
      }
      frame "Target Timeout Error" {
        w153 = 42 items=["No error", "Argument error", "Memory is full", "Out of zone", "End of file", "File already open", "Generic file I/O error", "File not found", "File permission error", "Disk is full", "Duplicate path", "Too many files open", "System feature not enabled", "Resource file not found", "Cannot add resource", "Resource not found", "Image not found", "Image memory error", "Pen does not exist", "Config type invalid", "Config token not found", "Config parse error", "Config memory error", "Bad external code format", "Bad external code offset", "External code not present", "Null window", "Destroy window error", "Null menu", "Print aborted", "Bad print record", "Print driver error", "Windows error during printing", "Memory error during printing", "Print dialog error", "Generic print error", "Invalid device refnum", "Device not found", "Device parameter error", "Device unit error", "Cannot open device", "Device call aborted", "Generic error", "Cancelled by user", "Object ID too low", "Object ID too high", "Object not in heap", "Unknown heap", "Unknown object (invalid DefProc)", "Unknown object (DefProc not in table)", "Message out of range", "Invalid (null) method", "Unknown message", "Manager call not supported", "Bad address", "Network operation in progress", "Network operation timed out", "Connection is busy", "Network attribute not supported", "Network error", "Address in use", "System out of memory", "Connection aborted", "Connection refused", "Not connected", "Already connected", "Connection closed", "Initialization error (interapplication manager)", "Bad occurrence", "Wait on unbound occurrence handler", "Occurrence queue overflow", "Datalog type conflict", "Unused", "Unrecognized type (interapplication manager)", "Memory corrupt", "Failed to make temporary DLL", "Old CIN version", "Drag socket not found", "Failed to load drop-object", "Failed to register OLE object", "Failed to release OLE object", "Format specifier type mismatch", "Unknown format specifier", "Too few format specifiers", "Too many format specifiers", "Scan failed", "Newer CIN version", "Error converting to variant", "Runtime menu error", "Password tampered", "Variant attribute not found", "Incompatible variant data type", "Event data is not available", "Event Store is not present", "Occurrence is not found", "Event Queue is not created", "Event info is not available", "Refnum passed is NULL", "Error retrieving Class GUID", "Error retrieving CoClass GUID", "Error retrieving TypeLib GUID.", "Bad built application magic bytes.", "Specific driver is different from the specific driver associated with the Logical Name.", "There is no session opened to the class driver.", "Max Error", "MAX - Error with config objects", "MAX - Error loading configuration", "MAX - Group not supported"]
        # "Handle target timeout error here.\nWhen this CSM could not get the sync-call response in time, this CSM goes into this case."
        # "Handle mistyped state name (developer tool)"
        n43 = Format Into String(format string="Software Exception: Target could not finish the \"%s\" state in time." ("message"), error in=w150, w145) -> (resulting string=w152:string, error out=w151:errorcluster)  [unwired: 1 in]
        n44 = call <vilib>:"Error Cluster From Error Code.vi"("show call chain? (False)"=TRUE, "error in (no error)"=w151, "error message (\"\")"=w152, "error code (0)"=w153) -> ("error out"=w142:errorcluster)  [unwired: 5 in]
        n45 = call <vilib>:"General Error Handler.vi"("error in (no error)"=w142) -> ()  [unwired: 10 in, 5 out]
        n46 = call <vilib>:"Add State(s) to Queue__JKI_lib_State_Machine.vi"("State(s) in (\"\")"=w149) -> ("States Out"=w148:string)  [unwired: 14 in]
      }
      frame "Target Error" {
        w166 = 42 items=["No error", "Argument error", "Memory is full", "Out of zone", "End of file", "File already open", "Generic file I/O error", "File not found", "File permission error", "Disk is full", "Duplicate path", "Too many files open", "System feature not enabled", "Resource file not found", "Cannot add resource", "Resource not found", "Image not found", "Image memory error", "Pen does not exist", "Config type invalid", "Config token not found", "Config parse error", "Config memory error", "Bad external code format", "Bad external code offset", "External code not present", "Null window", "Destroy window error", "Null menu", "Print aborted", "Bad print record", "Print driver error", "Windows error during printing", "Memory error during printing", "Print dialog error", "Generic print error", "Invalid device refnum", "Device not found", "Device parameter error", "Device unit error", "Cannot open device", "Device call aborted", "Generic error", "Cancelled by user", "Object ID too low", "Object ID too high", "Object not in heap", "Unknown heap", "Unknown object (invalid DefProc)", "Unknown object (DefProc not in table)", "Message out of range", "Invalid (null) method", "Unknown message", "Manager call not supported", "Bad address", "Network operation in progress", "Network operation timed out", "Connection is busy", "Network attribute not supported", "Network error", "Address in use", "System out of memory", "Connection aborted", "Connection refused", "Not connected", "Already connected", "Connection closed", "Initialization error (interapplication manager)", "Bad occurrence", "Wait on unbound occurrence handler", "Occurrence queue overflow", "Datalog type conflict", "Unused", "Unrecognized type (interapplication manager)", "Memory corrupt", "Failed to make temporary DLL", "Old CIN version", "Drag socket not found", "Failed to load drop-object", "Failed to register OLE object", "Failed to release OLE object", "Format specifier type mismatch", "Unknown format specifier", "Too few format specifiers", "Too many format specifiers", "Scan failed", "Newer CIN version", "Error converting to variant", "Runtime menu error", "Password tampered", "Variant attribute not found", "Incompatible variant data type", "Event data is not available", "Event Store is not present", "Occurrence is not found", "Event Queue is not created", "Event info is not available", "Refnum passed is NULL", "Error retrieving Class GUID", "Error retrieving CoClass GUID", "Error retrieving TypeLib GUID.", "Bad built application magic bytes.", "Specific driver is different from the specific driver associated with the Logical Name.", "There is no session opened to the class driver.", "Max Error", "MAX - Error with config objects", "MAX - Error loading configuration", "MAX - Group not supported"]
        # "Handle target error here.\nWhen this CSM try to communicate with an un-existed CSM, this CSM goes into this case."
        # "Handle mistyped state name (developer tool)"
        n47 = Format Into String(format string="Software Exception: Target \"%s\" does not exists." ("message"), error in=w163, w158) -> (resulting string=w165:string, error out=w164:errorcluster)  [unwired: 1 in]
        n48 = call <vilib>:"Error Cluster From Error Code.vi"("show call chain? (False)"=TRUE, "error in (no error)"=w164, "error message (\"\")"=w165, "error code (0)"=w166) -> ("error out"=w156:errorcluster)  [unwired: 5 in]
        n49 = call <vilib>:"General Error Handler.vi"("error in (no error)"=w156) -> ()  [unwired: 10 in, 5 out]
        n50 = call <vilib>:"Add State(s) to Queue__JKI_lib_State_Machine.vi"("State(s) in (\"\")"=w162) -> ("States Out"=w161:string)  [unwired: 14 in]
      }
      frame "Async Response", "Response" {
        # "Handle Async-call Response (\"Async Response\" for ->)"
        # "Handle Sync-call Response (\"Response\" for -@)"
        # "After Message is executed, CSM+ goes to this state for receive the response. \n    For Async Message(->), \"Async Response\" is used. This CSM will goes to \"Async Message Posted\" immediately and receive the \"Async Response\" after the callee finishes the message.\n    For Sync Message(@),  This CSM will wait until the message is done and immediately goes to \"Response\""
      }
      frame "Async Message Posted" {
        # "Handle post action for async message (->)."
        # "After Async Message is posted (->), CSM+ goes to this state for post-action. You can use Argument - State to tell which Async Message is called."
      }
      frame "Initialize Core Data" {
        # "Do not delete, rename, or modify this frame.\n(this is used to determine panel behavior on exit)"
        # "originally closed?"
        # "exe?"
        # "If panel starts closed or is an EXE, then close it when we exit"
        n51 = property class="VI"() -> ("FP.State"=w179:T1)  [unwired: 2 in, 2 out]
        n52 = property class="App"() -> ("App.Kind"=w185:T2)  [unwired: 2 in, 2 out]
        n53 = control-ref of="Current VI Reference"() -> (w180:refnum<vi>)
        n54 = Equal?(x=w179, y=T1."Closed" ("Front Panel Window:State")) -> (x = y?=w177:bool)
        n55 = Equal?(x=w185, y=T2."Run Time System" ("Application:Kind")) -> (x = y?=w183:bool)
        n56 = Or(x=w177, y=w183) -> (x .or. y?=w181:bool)
        n57 = Bundle By Name(cluster=w182, "Core.Current VI Reference"=w180, "Core.Close Panel on Exit?"=w181) -> (w187:T9)
        n58 = call <vilib>:"Add State(s) to Queue__JKI_lib_State_Machine.vi"("State(s) in (\"\")"=w189) -> ("States Out"=w188:string)  [unwired: 14 in]
      }
      frame "Exit" {
        # "Do not put any code in this frame.\n(No errors that occur here will be handled.)"
        n59 = local write "Status"("Exit" ("Exit String")) -> ()
        n60 = call <vilib>:"Add State(s) to Queue__JKI_lib_State_Machine.vi"("State(s) in (\"\")"=w196) -> ("States Out"=w195:string)  [unwired: 14 in]
      }
      frame "---------- Data ----------" {
        # "Do not put any code in this frame.\n(It is a separator no-op. You can make a copy of this frame to create a new Data frame)"
        n61 = call <vilib>:"Add State(s) to Queue__JKI_lib_State_Machine.vi"("State(s) in (\"\")"=w201) -> ("States Out"=w200:string)  [unwired: 14 in]
      }
      frame "Data: Initialize" {
        w210 = UI_State."Idle"  # State
        w211 = T8 {"Start Ref"=refnum, "Stop Ref"=refnum, "Settings Ref"=refnum, "Exit Ref"=refnum, "Status Ref"=refnum, "Data Ref"=refnum}  # UI Refs
        w209 = T4 {"Hardware"={"Resource"="", "SignalType"=enum."Sine Wave"}, "Logging"={"BasePath"=path ""}}  # Config
        w213 = T10 {"Current VI Reference"=refnum, "Close Panel on Exit?"=FALSE}  # Core
        # "Initialize the shift-register data, here.\n(data names are defined by what you wire into the bundle function)"
        n62 = call <userlib>:"CSM - Config MassData Parameter Cache Size.vi"("Error in"=w203, "size(1M)"=100000000) -> ("Error out"=w202:errorcluster)  [unwired: 9 in]
        n63 = call <vilib>:"Application Directory.vi"() -> ("Application Directory"=w206:path)
        n64 = Build Path(base path=w206, name or relative path=path "_data") -> (appended path=w207:path)
        n65 = Bundle By Name(cluster=w209, "Logging.BasePath"=w207) -> (w204:T4)
        n66 = Bundle("Core"=w213, "Config"=w204, "UI Refs"=w211, "State"=w210) -> (w214:T9)  [unwired: 1 in]
        n67 = call <vilib>:"Add State(s) to Queue__JKI_lib_State_Machine.vi"("State(s) in (\"\")"=w216) -> ("States Out"=w215:string)  [unwired: 14 in]
      }
      frame "Data: Load Configuration From Ini" {
        n68 = call <userlib>:"CSM - Populate Configuration Variables.vi"("String in"="Data: Set Configuration >> Config.Hardware.Resource:${Hardware.Resource}\nData: Set Configuration >> Config.Hardware.SignalType:${Hardware.SignalType:Sine Wave}\nData: Set Configuration >> Config.Logging.BasePath:${Logging.BasePath:C:\\data}" ("State(s) in Front (\"\")")) -> ("String out"=w218:string)  [unwired: 7 in, 1 out]
        n69 = call <vilib>:"Add State(s) to Queue__JKI_lib_State_Machine.vi"("State(s) in Front (\"\")"=w218, "State(s) in (\"\")"=w220) -> ("States Out"=w219:string)  [unwired: 13 in]
      }
      frame "Data: Save Configuration to Ini" {
        n70 = Unbundle By Name(w232) -> ("Config"=w231:T4)
        n71 = call "Convert Data To API String Arguments.vim"("data"=w231) -> ("String"=w230:string)  [unwired: 7 in, 1 out]
        n72 = Match Pattern(string=w230, regular expression="{") -> (after substring=w228:string)  [unwired: 1 in, 3 out]
        n73 = call <userlib>:"Default Ini Config File.vi"() -> ("appended path"=w237:path)  [unwired: 11 in]
        n74 = Match Pattern(string=w228, regular expression="}") -> (before substring=w226:string)  [unwired: 1 in, 3 out]
        n75 = call <userlib>:"String to 1D Array__ogtk.vi"("delimiter (Tab)"=";", "string"=w226) -> ("Array of Strings"=w224:string[])  [unwired: 9 in]
        n76 = call <userlib>:"Open.vi"("Create if not exists? (T)"=FALSE, "Path"=w237) -> ("error out"=w235:errorcluster, "Config"=w236:T11)  [unwired: 6 in, 2 out]
        n77 = for {
          shift-right: [w250] -> w234
          shift-left: w236 -> [w252]
          shift-right: [w249] -> w233
          shift-left: w235 -> [w251]
          tunnel: w224 -> [w248] mode=indexing
          n78 = Match Pattern(string=w248, regular expression=":") -> (before substring=w245:string, after substring=w246:string)  [unwired: 1 in, 2 out]
          n79 = Match Pattern(string=w245, regular expression="[.]") -> (before substring=w242:string, after substring=w243:string)  [unwired: 1 in, 2 out]
          n80 = call-poly <userlib>:"Write Key.vi"("Section Name"=w242, "error in (no error)"=w251, "Value"=w246, "Key Name"=w243, "Config in"=w252) -> ("error out"=w249:errorcluster, "Config out"=w250:T11)  [unwired: 4 in, 1 out]
        }
        n81 = call <userlib>:"Close.vi"("error in (no error)"=w233, "Config"=w234) -> ()  [unwired: 8 in, 2 out]
      }
      frame "Data: Set Configuration" {
        n82 = call "Convert API String Arguments to Data.vim"("Type"=w255, "String"=w256) -> ("error"=w253:errorcluster, "Data"=w254:T9)  [unwired: 6 in]
      }
      frame "Data: Get Configuration", "Data: Get Internal Data" {
        n83 = call "Query Data as API String Arguments.vim"("Setting Name"=w262, "Internal Data"=w263) -> ("error"=w261:errorcluster, "Setting as String"=w260:string, "Internal Data(dup)"=w259:T9)  [unwired: 7 in]
      }
      frame "Data: Cleanup" {
        # "Cleanup any data and references, here.\n(this is called automatically, by the Macro: Exit)"
        n84 = Unbundle By Name(w267) -> ("Core.Current VI Reference"=w270:refnum<vi>)
        n85 = Close Reference(reference=w270, error in (no error)=w269) -> (error out=w268:errorcluster)
        n86 = call <vilib>:"Add State(s) to Queue__JKI_lib_State_Machine.vi"("State(s) in (\"\")"=w272) -> ("States Out"=w271:string)  [unwired: 14 in]
      }
      frame "---------- Events ----------" {
        # "Do not put any code in this frame.\n(It is a separator no-op. You can make a copy of this frame to create a new UI frame)"
        n87 = call <vilib>:"Add State(s) to Queue__JKI_lib_State_Machine.vi"("State(s) in (\"\")"=w277) -> ("States Out"=w276:string)  [unwired: 14 in]
      }
      frame "Events: Register" {
        # "Register message event to break Waiting in Event structure."
        n88 = call <userlib>:"CSM - Get New State Notifier Event.vi"("Name(\"\" to use uuid) in"=w280) -> ("Error out"=w278:errorcluster, "New State Notifier Event"=w279:refnum<user-event>)  [unwired: 9 in]
        n89 = register-events(w279) -> (reference out=w281:refnum<event-registration>)  [unwired: 2 in, 1 out]
      }
      frame "Events: Unregister" {
        n90 = Unregister For Events(event registration refnum=w284, error in=w288) -> (error out=w285:errorcluster)
      }
      frame "---------- UI ----------" {
        # "Do not put any code in this frame.\n(It is a separator no-op. You can make a copy of this frame to create a new UI frame)"
        n91 = call <vilib>:"Add State(s) to Queue__JKI_lib_State_Machine.vi"("State(s) in (\"\")"=w293) -> ("States Out"=w292:string)  [unwired: 14 in]
      }
      frame "UI: Initialize" {
        # "Initialize the User Interface, here.\n(this is called automatically, by the Macro: Init)"
        n92 = control-ref of="Data"() -> (w299:refnum<vi>)
        n93 = control-ref of="Start"() -> (w304:refnum<vi>)
        n94 = control-ref of="Stop"() -> (w303:refnum<vi>)
        n95 = control-ref of="Settings"() -> (w305:refnum<vi>)
        n96 = control-ref of="Exit"() -> (w306:refnum<vi>)
        n97 = control-ref of="Status"() -> (w300:refnum<vi>)
        n98 = Bundle By Name(cluster=w296, "UI Refs.Start Ref"=w304, "UI Refs.Stop Ref"=w303, "UI Refs.Settings Ref"=w305, "UI Refs.Exit Ref"=w306, "UI Refs.Status Ref"=w300, "UI Refs.Data Ref"=w299) -> (w295:T9)
        n99 = Build Array(w304, w306, w305) -> (w302:refnum<vi>[])
        n100 = Build Array(w303) -> (w301:refnum<vi>[])
        n101 = property on="Data" class="WFChart (strict)"("History Data"=waveform(dbl)[][] []) -> ()  [unwired: 2 in, 2 out]
        n102 = call "Set Enable State on Multiple Controls.vi"("Enable?"=TRUE, "Controls"=w302) -> ()  [unwired: 10 in]
        n103 = call "Set Enable State on Multiple Controls.vi"("Enable?"=FALSE, "Controls"=w301) -> ()  [unwired: 10 in]
        n104 = call <vilib>:"Add State(s) to Queue__JKI_lib_State_Machine.vi"("State(s) in (\"\")"=w310) -> ("States Out"=w309:string)  [unwired: 14 in]
      }
      frame "UI: Update When Start" {
        # "Enable: Stop\nDisable: Start, Exit, Settings"
        n105 = Unbundle By Name(w311) -> ("UI Refs.Stop Ref"=w317:refnum<vi>, "UI Refs.Start Ref"=w316:refnum<vi>, "UI Refs.Exit Ref"=w315:refnum<vi>, "UI Refs.Settings Ref"=w314:refnum<vi>)
        n106 = Build Array(w316, w315, w314) -> (w319:refnum<vi>[])
        n107 = Build Array(w317) -> (w318:refnum<vi>[])
        n108 = call "Set Enable State on Multiple Controls.vi"("Enable?"=TRUE, "Controls"=w318) -> ()  [unwired: 10 in]
        n109 = call "Set Enable State on Multiple Controls.vi"("Enable?"=FALSE, "Controls"=w319) -> ()  [unwired: 10 in]
      }
      frame "UI: Update When Stop" {
        # "Enable: Start, Exit, Settings\nDisable: Stop"
        n110 = Unbundle By Name(w323) -> ("UI Refs.Stop Ref"=w328:refnum<vi>, "UI Refs.Start Ref"=w329:refnum<vi>, "UI Refs.Exit Ref"=w330:refnum<vi>, "UI Refs.Settings Ref"=w331:refnum<vi>)
        n111 = Build Array(w329, w330, w331) -> (w326:refnum<vi>[])
        n112 = Build Array(w328) -> (w327:refnum<vi>[])
        n113 = call "Set Enable State on Multiple Controls.vi"("Enable?"=FALSE, "Controls"=w327) -> ()  [unwired: 10 in]
        n114 = call "Set Enable State on Multiple Controls.vi"("Enable?"=TRUE, "Controls"=w326) -> ()  [unwired: 10 in]
      }
      frame "UI: Cursor Set" {
        # "Argument"
        # "Set and Unset Cursor Busy.\n(Usage: \"UI: Cursor Set >> Busy|Idle\")"
        n115 = disable-structure shown="TARGET_TYPE!=Windows" {
          disable-tunnel: w338 -> [w344 w349]
          disable-tunnel: [w343 w349] -> w337
          disable-tunnel: w336 -> [w342 _]
          frame condition #0 (active) {
            n116 = case shown="\"Busy\"" w342 {
              tunnel: w344 -> [w346 w348]
              tunnel: [w345 w347] -> w343
              frame "Idle", Default {
                n117 = call <vilib>:"Unset Busy.vi"("error in (no error)"=w346) -> ("error out"=w345:errorcluster)  [unwired: 10 in]
              }
              frame "Busy" {
                n118 = call <vilib>:"Set Busy.vi"("error in (no error)"=w348) -> ("error out"=w347:errorcluster)  [unwired: 9 in, 1 out]
              }
            }
          }
          frame condition #1 {
          }
        }
        n119 = call <vilib>:"Add State(s) to Queue__JKI_lib_State_Machine.vi"("State(s) in (\"\")"=w341) -> ("States Out"=w340:string)  [unwired: 14 in]
      }
      frame "UI: Front Panel State" {
        # "Argument"
        # "Set Front Panel Open or Closed\n(Usage: \"UI: Front Panel State >> Open|Close\")"
        n120 = Unbundle By Name(w353) -> ("Core.Current VI Reference"=w352:refnum<vi>)
        n121 = case shown="\"Minimize\", \"Minimized\"" w351 {
          tunnel: w355 -> [w363 w378 w389 w402 w415]
          tunnel: [w365 w379 w391 w404 w417] -> w354
          tunnel: w352 -> [w364 w376 w390 w403 w416]
          frame "Open", "Standard", Default {
            w358 = T1."Standard" ("State")
            n122 = property class="VI"(reference=w364, error in=w363) -> (reference out=w361:refnum<vi>, error out=w362:errorcluster, "FP.State"=w360:T1)
            n123 = Not Equal?(x=w360, y=w358) -> (x != y?=w359:bool)
            n124 = case shown="True" w359 {
              tunnel: [w369 w371] -> w365
              tunnel: w362 -> [w368 w371]
              tunnel: w361 -> [w367 _]
              tunnel: w358 -> [w366 _]
              frame True {
                n125 = invoke class="VI" method="FP.Open"(reference=w367, error in=w368, "Activate"=TRUE, "State"=w366) -> (error out=w369:errorcluster)  [unwired: 1 in, 4 out]
              }
              frame False {
              }
            }
          }
          frame "Close", "Closed" {
            n126 = property class="VI"(reference=w376, error in=w378) -> (reference out=w375:refnum<vi>, error out=w377:errorcluster, "FP.State"=w373:T1)
            n127 = Not Equal?(x=w373, y=T1."Closed" ("Front Panel Window:State")) -> (x != y?=w372:bool)
            n128 = case shown="True" w372 {
              tunnel: [w380 w383] -> w379
              tunnel: w377 -> [w380 w382]
              tunnel: w375 -> [_ w381]
              frame False {
              }
              frame True {
                n129 = invoke class="VI" method="FP.Close"(reference=w381, error in=w382) -> (error out=w383:errorcluster)  [unwired: 1 in, 2 out]
              }
            }
          }
          frame "Hidden", "Hide" {
            w384 = T1."Hidden" ("State")
            n130 = property class="VI"(reference=w390, error in=w389) -> (reference out=w387:refnum<vi>, error out=w388:errorcluster, "FP.State"=w386:T1)
            n131 = Not Equal?(x=w386, y=w384) -> (x != y?=w385:bool)
            n132 = case shown="True" w385 {
              tunnel: [w395 w396] -> w391
              tunnel: w388 -> [w394 w396]
              tunnel: w387 -> [w393 _]
              tunnel: w384 -> [w392 _]
              frame True {
                n133 = invoke class="VI" method="FP.Open"(reference=w393, error in=w394, "State"=w392) -> (error out=w395:errorcluster)  [unwired: 2 in, 4 out]
              }
              frame False {
              }
            }
          }
          frame "Minimize", "Minimized" {
            w397 = T1."Minimized" ("State")
            n134 = property class="VI"(reference=w403, error in=w402) -> (reference out=w400:refnum<vi>, error out=w401:errorcluster, "FP.State"=w399:T1)
            n135 = Not Equal?(x=w399, y=w397) -> (x != y?=w398:bool)
            n136 = case shown="True" w398 {
              tunnel: [w408 w409] -> w404
              tunnel: w401 -> [w407 w409]
              tunnel: w400 -> [w406 _]
              tunnel: w397 -> [w405 _]
              frame True {
                n137 = invoke class="VI" method="FP.Open"(reference=w406, error in=w407, "State"=w405) -> (error out=w408:errorcluster)  [unwired: 2 in, 4 out]
              }
              frame False {
              }
            }
          }
          frame "Maximize", "Maximized" {
            w410 = T1."Maximized" ("State")
            n138 = property class="VI"(reference=w416, error in=w415) -> (reference out=w413:refnum<vi>, error out=w414:errorcluster, "FP.State"=w412:T1)
            n139 = Not Equal?(x=w412, y=w410) -> (x != y?=w411:bool)
            n140 = case shown="True" w411 {
              tunnel: [w421 w422] -> w417
              tunnel: w414 -> [w420 w422]
              tunnel: w413 -> [w419 _]
              tunnel: w410 -> [w418 _]
              frame True {
                n141 = invoke class="VI" method="FP.Open"(reference=w419, error in=w420, "State"=w418) -> (error out=w421:errorcluster)  [unwired: 2 in, 4 out]
              }
              frame False {
              }
            }
          }
        }
        n142 = call <vilib>:"Add State(s) to Queue__JKI_lib_State_Machine.vi"("State(s) in (\"\")"=w357) -> ("States Out"=w356:string)  [unwired: 14 in]
      }
      frame "UI: Update Waveforms" {
        n143 = call "CSM - Convert Argument to MassData.vim"("Type"=waveform(dbl)[] [] ("Data"), "HEX Argument"=w426) -> ("error out"=w423:errorcluster, "DBL"=→"Data":waveform(dbl)[])  [unwired: 6 in]
      }
      frame "---------- Macro ----------" {
        # "Do not put any code in this frame.\n(It is a separator no-op. You can make a copy of this frame to create a new Macro frame)"
        n144 = call <vilib>:"Add State(s) to Queue__JKI_lib_State_Machine.vi"("State(s) in (\"\")"=w434) -> ("States Out"=w433:string)  [unwired: 14 in]
      }
      frame "Macro: Initialize" {
        # "Initialization Macro\n(This is called once, when the VI starts)"
        n145 = disable-structure "Diagram Disable Structure" shown="Disabled" {
          frame Disabled {
            # "Acquired Waveform@Acquisition >> UI: Update Waveforms -><register>"
            n146 = call <userlib>:"CSM - Register Status Change.vi"("CSM Name"="UI", "Source CSM Name (* as Default)"="Acquisition", "Status"="Acquired Waveform" ("Source CSM Name (* as Default)"), "Response Message (if \"\", same as Source Message)"="UI: Update Waveforms" ("Source CSM Name (* as Default)")) -> ()  [unwired: 10 in, 2 out]
          }
          frame Enabled {
          }
        }
        n147 = call <userlib>:"CSM - Populate Configuration Variables.vi"("String in"="Data: Initialize\nInitialize Core Data\nData: Load Configuration From Ini\nEvents: Register\nUI: Initialize\nUI: Front Panel State >> Open\nDo: Update Settings\nDO: Update Status >> Ready...\n//Same as code in Diagram Disable Structure below\nAcquired Waveform@Acquisition >> UI: Update Waveforms -><register>") -> ("String out"=w436:string)  [unwired: 7 in, 1 out]
        n148 = call <vilib>:"Add State(s) to Queue__JKI_lib_State_Machine.vi"("State(s) in Front (\"\")"=w436, "State(s) in (\"\")"=w441) -> ("States Out"=w440:string)  [unwired: 13 in]
      }
      frame "Macro: Start" {
        n149 = disable-structure shown="Disabled" {
          frame Disabled {
            # "Acquired Waveform@Acquisition >> API: Log@Logging -><register>"
            n150 = call <userlib>:"CSM - Register Status Change.vi"("CSM Name"="Logging", "Source CSM Name (* as Default)"="Acquisition", "Status"="Acquired Waveform" ("Source CSM Name (* as Default)"), "Response Message (if \"\", same as Source Message)"="API: Log" ("Source CSM Name (* as Default)")) -> ()  [unwired: 10 in, 2 out]
          }
          frame Enabled {
          }
        }
        n151 = call <vilib>:"Add State(s) to Queue__JKI_lib_State_Machine.vi"("State(s) in Front (\"\")"="//Same as code in Diagram Disable Structure below\nAcquired Waveform@Acquisition >> API: Log@Logging -><register>\nDO: Update Status >> Acquiring and Logging...\nUI: Update When Start\nAPI: Start ->| Logging\nAPI: Start ->| Acquisition" ("State(s) in Front (\"\")"), "State(s) in (\"\")"=w447) -> ("States Out"=w448:string)  [unwired: 13 in]
        n152 = Bundle By Name(cluster=w450, "State"=UI_State."Acquiring and Logging" ("UI State")) -> (w449:T9)
      }
      frame "Macro: Stop" {
        n153 = disable-structure shown="Disabled" {
          frame Disabled {
            # "Acquired Waveform@Acquisition >> *@Logging -><unregister>"
            n154 = call <userlib>:"CSM - Unregister Status Change.vi"("CSM Name"="Logging", "Source CSM Name"="Acquisition" ("Source CSM Name (* as Default)"), "Status"="Acquired Waveform" ("Source CSM Name (* as Default)")) -> ()  [unwired: 11 in, 2 out]
          }
          frame Enabled {
          }
        }
        n155 = Unbundle By Name(w458) -> ("State"=w460:T3)
        n156 = case shown="Default" w460 {
          selector: w460 -> [w470 _]
          tunnel: [w470 UI_State."Waiting for Stop" ("UI State")] -> w459
          frame "Waiting for Exit" {
          }
          frame Default {
          }
        }
        n157 = Bundle By Name(cluster=w458, "State"=w459) -> (w464:T9)
        n158 = call <vilib>:"Add State(s) to Queue__JKI_lib_State_Machine.vi"("State(s) in Front (\"\")"="DO: Update Status >> Stoping...\nUI: Update When Stop\nAPI: Stop ->| Logging\nAPI: Stop ->| Acquisition\n//Same as code in Diagram Disable Structure below\nAcquired Waveform@Acquisition >> *@Logging -><unregister>" ("State(s) in Front (\"\")"), "State(s) in (\"\")"=w462) -> ("States Out"=w463:string)  [unwired: 13 in]
      }
      frame "Macro: Exit" {
        # "Exit Macro\n(This is called once, when the VI exits)"
        n159 = Unbundle By Name(w480) -> ("Core.Close Panel on Exit?"=w479:bool)
        n160 = Select(t="UI: Front Panel State >> Close", s=w479, f="") -> (s? t:f=w476:string)
        n161 = call <vilib>:"Add State(s) to Queue__JKI_lib_State_Machine.vi"("State(s) in Front (\"\")"="Macro: Exit -@ Acquisition\nMacro: Exit -@ Logging\nMacro: Exit -@ Algorithm", "State(s) in (\"\")"=w476, "State(s) at Back (\"\")"="Data: Save Configuration to Ini\nData: Cleanup\nEvents: Unregister\nExit") -> ("States Out"=w474:string)  [unwired: 12 in]
        n162 = call <vilib>:"Add State(s) to Queue__JKI_lib_State_Machine.vi"("State(s) in Front (\"\")"=w474, "State(s) in (\"\")"=w483) -> ("States Out"=w482:string)  [unwired: 13 in]
      }
      frame "---------- DoSth ----------" {
        # "Template Separator\n(You can make a copy of, or modify, this frame)"
        n163 = call <vilib>:"Add State(s) to Queue__JKI_lib_State_Machine.vi"("State(s) in (\"\")"=w488) -> ("States Out"=w487:string)  [unwired: 14 in]
      }
      frame "Do: Update Status" {
        # "Your code here.\n(You can make a copy of, or modify, this frame)"
        n164 = call <vilib>:"Add State(s) to Queue__JKI_lib_State_Machine.vi"("State(s) in (\"\")"=w494) -> ("States Out"=w493:string)  [unwired: 14 in]
        "Status" <- w489
      }
      frame "Do: Launch Settings Dialog" {
        # "Your code here.\n(You can make a copy of, or modify, this frame)"
        n165 = Unbundle By Name(w500) -> ("Config"=w502:T4)
        n166 = call-by-ref "?"("error in (no error)"=w498, "Settings in"=w502) -> ("error out"=w497:errorcluster, "Cancelled?"=w496:bool, "Settings out"=w501:T4)  [unwired: 8 in, 3 out]
        n167 = Bundle By Name(cluster=w500, "Config"=w501) -> (w499:T9)
        n168 = call-poly <userlib>:"Add State(s) to Queue By BOOL++.vi"("False(\"\")"="Do: Update Settings" ("False(\"\")"), "Bool"=w496, "State Queue(\"\")"=w505) -> ("State Queue Out"=w504:string)  [unwired: 8 in]
      }
      frame "Do: Update Settings" {
        w509 = "API: Update Settings" ("State")
        n169 = Unbundle By Name(w516) -> ("Config.Logging.BasePath"=w515:path, "Config.Hardware"=w513:T5)
        n170 = Path To String(path=w515) -> (string=w514:string)
        n171 = call <userlib>:"CSM - Convert Data to HexStr.vi"("Variant"=w513) -> ("HEX String (0-9,A-F)"=w510:string)  [unwired: 8 in]
        n172 = call-poly <userlib>:"Build Message with Arguments++.vi"("State with Arguments"=w509, "Arguments (\"\")"=w514, "Target Module (\"\")"="Logging" ("Target Module (\"\")")) -> ("State with Arguments"=w508:string)  [unwired: 12 in]
        n173 = call-poly <userlib>:"Build Message with Arguments++.vi"("State with Arguments"=w509, "Arguments (\"\")"=w510, "Target Module (\"\")"="Acquisition" ("Target Module (\"\")")) -> ("State with Arguments"=w507:string)  [unwired: 12 in]
        n174 = call <vilib>:"Add State(s) to Queue__JKI_lib_State_Machine.vi"("State(s) in Front (\"\")"=w508, "State(s) in (\"\")"=w507) -> ("States Out"=w506:string)  [unwired: 13 in]
        n175 = call <vilib>:"Add State(s) to Queue__JKI_lib_State_Machine.vi"("State(s) in Front (\"\")"=w506, "State(s) in (\"\")"=w517) -> ("States Out"=w518:string)  [unwired: 13 in]
      }
      frame "Do: Confirm Quit" {
        n176 = Unbundle By Name(w527) -> ("State"=w530:T3)
        n177 = case shown="\"Acquiring and Logging\"" w530 {
          tunnel: [w535 w542] -> w525
          tunnel: [UI_State."Idle" ("UI State") w541] -> w529
          tunnel: w526 -> [w535 w540]
          tunnel: w527 -> [w534 w539]
          tunnel: [w534 w538] -> w528
          tunnel: [TRUE w537] -> w521
          frame Default {
          }
          frame "Acquiring and Logging" {
            n178 = Two Button Dialog(message="Are you sure you want to quit while the acquisition is running?" ("Confirm Quit Message"), 1:"No" ("No"), 2:"Yes" ("Yes")) -> (T button?=w543:bool)
            n179 = case shown="True" w543 {
              tunnel: [w548 w552] -> w542
              tunnel: [UI_State."Acquiring and Logging" ("UI State") UI_State."Waiting for Exit" ("UI State")] -> w541
              tunnel: w540 -> [w548 w552]
              tunnel: w539 -> [w547 w551]
              tunnel: [w547 w551] -> w538
              tunnel: [_ TRUE] -> w537
              frame False {
                # "User did not want to quit."
              }
              frame True {
              }
            }
          }
        }
        n180 = Bundle By Name(cluster=w528, "State"=w529) -> (w524:T9)
        n181 = call-poly <userlib>:"Add State(s) to Queue By BOOL++.vi"("TRUE(\"\")"="Macro: Exit", "Bool"=w521, "State Queue(\"\")"=w532) -> ("State Queue Out"=w523:string)  [unwired: 8 in]
      }
    }
  }
  "error out" <- w4
  n182 = call "Acquisition.vi"("Name(\"\" to use uuid)"="Acquisition" ("Name(\"\" to use uuid)")) -> ()  [unwired: 11 in]
  n183 = call "Logging.vi"("Name(\"\" to use uuid)"="Logging" ("Name(\"\" to use uuid)")) -> ()  [unwired: 11 in]
  n184 = call "Algorithm.vi"("Name(\"\" to use uuid)"="Algorithm" ("Name(\"\" to use uuid)")) -> ()  [unwired: 11 in]
